vi "Menu Buttons.vi"(8 "error in (no error)":errorcluster, 10 "Valid/enable":bool, 11 "Data":T1) -> (0 "error out":errorcluster, 3 "Data Out":T1)   [LabVIEW 2019, in "SubVI.lvlib"]
uses:
  ATM/controls/Data.ctl
  ATM/controls/Message Type.ctl
  ATM/controls/ATM Action.ctl
  SubVI.lvlib
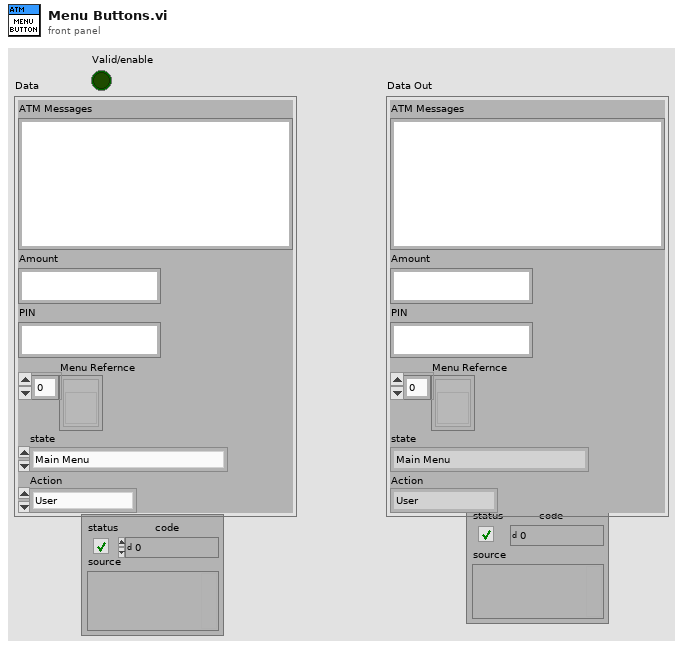
[diagram p1: front panel]
types:
  T1 = typedef "Data.ctl" = cluster{"ATM Messages":string, "Amount":string, "PIN":string, "Menu Refernce":refnum<vi>[], "state":T2, "Action":T3}
  T2 = typedef "Message Type.ctl" = enum16{"Main Menu", "Balance", "Withdrawal Complete", "Deposit Complete", "Welcome", "Account", "Session", "Deposit", "Withdraw", "Failed"}
  T3 = typedef "ATM Action.ctl" = enum16{"User", "Deposit", "Withdraw"}
  T4 = enum8{"Enabled", "Disabled", "Disabled and Grayed Out"}
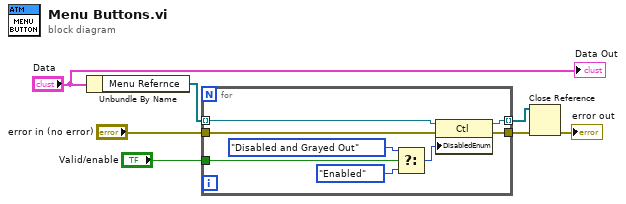
[diagram p0: block diagram]
diagram:
  n1 = Unbundle By Name("Data") -> ("Menu Refernce"=w5:refnum<vi>[])
  n2 = for {
    tunnel: "Valid/enable" -> [w11]
    tunnel: w5 -> [w12] mode=indexing
    tunnel: "error in (no error)" -> [w10]
    tunnel: [w9] -> w3 mode=indexing
    tunnel: [w8] -> w2
    n3 = Select(t=T4."Disabled and Grayed Out" ("Disabled"), s=w11, f=T4."Enabled" ("Disabled")) -> (s? t:f=w15:T4)
    n4 = property class="Ctl"(reference=w12, error in=w10, "DisabledEnum"=w15) -> (reference out=w9:refnum<vi>, error out=w8:errorcluster)
  }
  n5 = Close Reference(reference=w3, error in (no error)=w2) -> (error out=→"error out":errorcluster)
  "Data Out" <- "Data"
